vi "CSM - List Status in Broadcast Registry.vi"(8 "error in (no error)":errorcluster) -> (0 "error out":errorcluster, 3 "Broadcast Names":string[](array[string]))   [LabVIEW 2017, in "Communicable State Machine.lvlib"]
doc: "This VI is obsolete. Please use `CSM - List Sources in Broadcast Registry.vi`\n\n## CSM - List Sources in Broadcast Registry.vi\nLists the broadcast names of all current broadcast registration relationships.\n\n> - Ref: CSM Broadcast\n> - Ref: CSM Registration\n\n-- <b>Indicators</b> --\n- <b>Broadcast Names</b>: Broadcast names of all current broadcast registration relationships."
uses:
  Communicable State Machine.lvlib
  _Support/FGV-BroadcastRegistry/Operation-BroadcastRegistry.ctl
  _Support/ChangeFlag/ChangeFlag-Read.vi
  _Support/ChangeFlag/ChangeFlagDB.vi
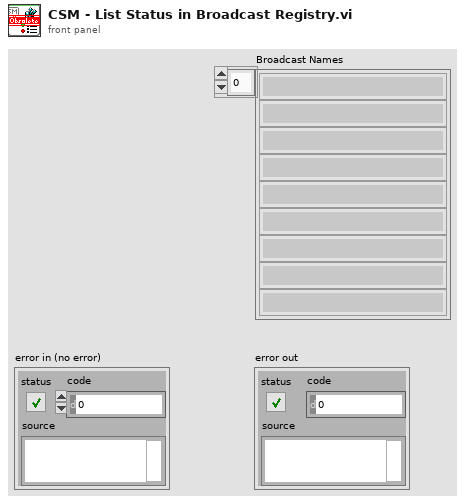
[diagram p1: front panel]
types:
  T1 = typedef "Communicable State Machine.lvlib/Operation-BroadcastRegistry.ctl" = enum16{"Delete Source Module", "Delete Target Module", "Remove Module", "Register", "Unregister", "Check", "List Status", "List Entries", "List Status Of Source", "Drop", "Register As Status", "Register As Interrupt"}
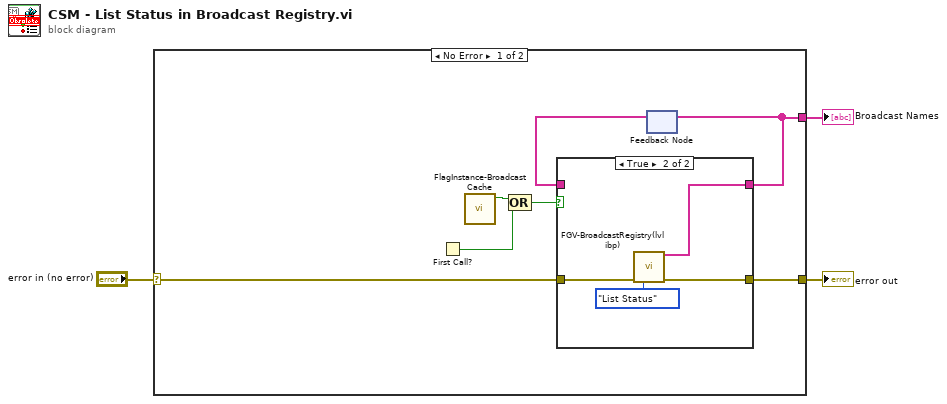
[diagram p0: block diagram]
diagram:
  n1 = case shown="No Error" "error in (no error)" {
    selector: "error in (no error)" -> [w10 w17]
    tunnel: [w7 _] -> w2
    tunnel: [w5 w17] -> w1
    frame No Error {
      n2 = First Call?() -> (First Call?: T/F=w9:bool)
      n3 = call "FlagInstance-Broadcast Cache.vi"() -> ("Changed"=w4:bool)  [unwired: 10 in, 1 out]
      n4 = Compound Arithmetic op=OR(w4, w9) -> (w8:bool)
      n5 = feedback #1() -> (w6:string[])  [unwired: 1 in]
      n6 = case shown="True" w8 {
        tunnel: [w12 w16] -> w5
        tunnel: w10 -> [w12 w15]
        tunnel: [w11 w13] -> w7
        tunnel: w6 -> [w11 _]
        frame False {
        }
        frame True {
          n7 = call "FGV-BroadcastRegistry(lvlibp).vi"("Error In"=w15, "Operation"=Operation-BroadcastRegistry."List Status") -> ("Response Message"=w13:string[], "error out"=w16:errorcluster)  [unwired: 11 in, 1 out]
        }
      }
      n8 = feedback-in #1(w7) -> ()
    }
    frame Error {
    }
  }
  "error out" <- w1
  "Broadcast Names" <- w2
